vi "ViperHawk_Decode Inv Data.vi"(9 "Washer In":T1={"Appliance Details"={"FileVersionInfo"={"FileVersion"="Version", "ProductName"="ProductName", "InternalName"="InternalName", "CompanyName"="CompanyName", "LegalCopyright"="LegalCopyright", "FileDescription"="FileDescription"}, "Dishwasher Info"={"Open Cup Weight (gm):"=0.0, "Auto Cup Weight (gm):"=0.0, "Detergent-Dish:"="", "Inlet Temperature-Dish:"="", "Cycle Mode-Dish:"="", "Unit Control-Dish:"="", "Manufacturer-Dish:"=""}, "Washer Info"={"Hot Water Temperature (Fahrenheit):"="", "Cold Water Temperature (Fahrenheit):"="", "Capacity (cu.ft):"=0.0, "Initial Cloth Weight:"=0.0, "Cloth Lot:"=0, "Model Family:"="", "Program Name:"="", "Cycle Selection:"="", "Wash Temperature:"="", "Rinse Temperature:"="", "Load Size:"=""}, "File Name Output Array"=[], "Calibration Output Array"=[], "Appliance Common"={"Engineer:"="", "Model Number:"="", "Serial Number:"="15HL2790", "Comments:"="", "Station ID:"="", "Technician:"="", "TR Number:"="15HL2790", "Lab ID:"="15HL2790", "Voltage:"="", "Water Pressure (PSI):"="", "Test Date:"="", "Computer Name:"="", "IP Address:"="", "Ambient RH:"="", "Frequency:"="", "Build:"="", "Filename:"="", "Test Type:"="", "Load Run #:"=0, "Ambient Temperature (F):"="", "File Path:"=path "", "Cycles Per Year"=60}, "Water Heater"={"Heating Mode:"=""}, "Dryer"={"Heat Setting:"="", "Washer Water Temperature (60 ± 5°F):"=60, "Water Hardness (PPM):"=17, "Dryness Setting:"="", "Dryer Type:"="", "Exhaust:"="", "Drying Cycle:"="", "Load Type:"="", "Nominal Load Weight"="", "Dryer Initial IMC Data"={"Measured IMC (lbs)"=7.0, "Actual Initial RMC (%)"=7.0, "RMC (Desired %)"=100.0, "Bone Dry Wt(lbs)"=7.0, "Tolerance(%)"=5.0, "Actual Final RMC (%)"=7.0, "CEF (lbf/kWh)"=0.0, "Minimum Weight (lbf)"=0.0, "Average Weight (lbf)"=0.0, "Maximum Weight (lbf)"=0.0, "Measured IMC In Range?"=FALSE, "Moisture Reduction Factor"=55.5, "Field Use Factor"=1.04, "Empty Dryer Cold Weigth"=0.0, "Energy Standard"=enum."D2-Automatic Dryer", "Weight Cloth (lbs)"=0.0, "Relative Moisture Content (%)"=0.0, "Relative Moisture Content - Avg (%)"=0.0}}}, "Display Data (RLT)"={"Status Color"=14927872, "Serial Number Display"="15HL2790", "Cycle Count Display"=0, "Station Label Display"="04125059", "Current Run Start Time Display"=0.0, "Board ID Display"="", "RPM Display"=0, "Current Display"=1.0, "Current Path Display"=path "", "Saving Display"=FALSE, "Unit Type Display"=enum."2015", "Total Time On Display"=0.0, "UI Button"=FALSE}} {"Display Data (RLT)"."Current Display" format="%.2f"; "Display Data (RLT)"."Cycle Count Display" format="%04d"; "Appliance Details"."Dryer"."Dryer Initial IMC Data"."Maximum Weight (lbf)" format="%03_6g"; "Appliance Details"."Dryer"."Dryer Initial IMC Data"."Average Weight (lbf)" format="%03_6g"; "Appliance Details"."Dryer"."Dryer Initial IMC Data"."Minimum Weight (lbf)" format="%03_6g"; "Appliance Details"."Dryer"."Dryer Initial IMC Data"."CEF (lbf/kWh)" format="%03_6g"; "Appliance Details"."Dryer"."Dryer Initial IMC Data"."Actual Final RMC (%)" format="%03_6g"; "Appliance Details"."Dryer"."Dryer Initial IMC Data"."Tolerance(%)" format="%0#_6g"; "Appliance Details"."Dryer"."Dryer Initial IMC Data"."Bone Dry Wt(lbs)" format="%03_6g"; "Appliance Details"."Dryer"."Dryer Initial IMC Data"."RMC (Desired %)" format="%0#_6g"; "Appliance Details"."Dryer"."Dryer Initial IMC Data"."Actual Initial RMC (%)" format="%03_6g"; "Appliance Details"."Dryer"."Dryer Initial IMC Data"."Measured IMC (lbs)" format="%0#_6g"}, 10 "Data":u8[](array[numeric]), 11 "Diagnostic Data In":T10) -> (1 "Washer Out":T1={"Appliance Details"={"FileVersionInfo"={"FileVersion"="Version", "ProductName"="ProductName", "InternalName"="InternalName", "CompanyName"="CompanyName", "LegalCopyright"="LegalCopyright", "FileDescription"="FileDescription"}, "Dishwasher Info"={"Open Cup Weight (gm):"=0.0, "Auto Cup Weight (gm):"=0.0, "Detergent-Dish:"="", "Inlet Temperature-Dish:"="", "Cycle Mode-Dish:"="", "Unit Control-Dish:"="", "Manufacturer-Dish:"=""}, "Washer Info"={"Hot Water Temperature (Fahrenheit):"="", "Cold Water Temperature (Fahrenheit):"="", "Capacity (cu.ft):"=0.0, "Initial Cloth Weight:"=0.0, "Cloth Lot:"=0, "Model Family:"="", "Program Name:"="", "Cycle Selection:"="", "Wash Temperature:"="", "Rinse Temperature:"="", "Load Size:"=""}, "File Name Output Array"=[], "Calibration Output Array"=[], "Appliance Common"={"Engineer:"="", "Model Number:"="", "Serial Number:"="15HL2790", "Comments:"="", "Station ID:"="", "Technician:"="", "TR Number:"="15HL2790", "Lab ID:"="15HL2790", "Voltage:"="", "Water Pressure (PSI):"="", "Test Date:"="", "Computer Name:"="", "IP Address:"="", "Ambient RH:"="", "Frequency:"="", "Build:"="", "Filename:"="", "Test Type:"="", "Load Run #:"=0, "Ambient Temperature (F):"="", "File Path:"=path "", "Cycles Per Year"=60}, "Water Heater"={"Heating Mode:"=""}, "Dryer"={"Heat Setting:"="", "Washer Water Temperature (60 ± 5°F):"=60, "Water Hardness (PPM):"=17, "Dryness Setting:"="", "Dryer Type:"="", "Exhaust:"="", "Drying Cycle:"="", "Load Type:"="", "Nominal Load Weight"="", "Dryer Initial IMC Data"={"Measured IMC (lbs)"=7.0, "Actual Initial RMC (%)"=7.0, "RMC (Desired %)"=100.0, "Bone Dry Wt(lbs)"=7.0, "Tolerance(%)"=5.0, "Actual Final RMC (%)"=7.0, "CEF (lbf/kWh)"=0.0, "Minimum Weight (lbf)"=0.0, "Average Weight (lbf)"=0.0, "Maximum Weight (lbf)"=0.0, "Measured IMC In Range?"=FALSE, "Moisture Reduction Factor"=55.5, "Field Use Factor"=1.04, "Empty Dryer Cold Weigth"=0.0, "Energy Standard"=enum."D2-Automatic Dryer", "Weight Cloth (lbs)"=0.0, "Relative Moisture Content (%)"=0.0, "Relative Moisture Content - Avg (%)"=0.0}}}, "Display Data (RLT)"={"Status Color"=14927872, "Serial Number Display"="15HL2790", "Cycle Count Display"=0, "Station Label Display"="04125059", "Current Run Start Time Display"=0.0, "Board ID Display"="", "RPM Display"=0, "Current Display"=1.0, "Current Path Display"=path "", "Saving Display"=FALSE, "Unit Type Display"=enum."2015", "Total Time On Display"=0.0, "UI Button"=FALSE}} {"Display Data (RLT)"."Current Display" format="%.2f"; "Display Data (RLT)"."Cycle Count Display" format="%04d"; "Appliance Details"."Dryer"."Dryer Initial IMC Data"."Maximum Weight (lbf)" format="%03_6g"; "Appliance Details"."Dryer"."Dryer Initial IMC Data"."Average Weight (lbf)" format="%03_6g"; "Appliance Details"."Dryer"."Dryer Initial IMC Data"."Minimum Weight (lbf)" format="%03_6g"; "Appliance Details"."Dryer"."Dryer Initial IMC Data"."CEF (lbf/kWh)" format="%03_6g"; "Appliance Details"."Dryer"."Dryer Initial IMC Data"."Actual Final RMC (%)" format="%03_6g"; "Appliance Details"."Dryer"."Dryer Initial IMC Data"."Tolerance(%)" format="%0#_6g"; "Appliance Details"."Dryer"."Dryer Initial IMC Data"."Bone Dry Wt(lbs)" format="%03_6g"; "Appliance Details"."Dryer"."Dryer Initial IMC Data"."RMC (Desired %)" format="%0#_6g"; "Appliance Details"."Dryer"."Dryer Initial IMC Data"."Actual Initial RMC (%)" format="%03_6g"; "Appliance Details"."Dryer"."Dryer Initial IMC Data"."Measured IMC (lbs)" format="%0#_6g"}, 2 "Value":u8 format="%.0x", 3 "Diagnostic Data Out":T10)   [LabVIEW 2016]
uses:
  Type Definitions/ViperHawk/ViperHawk Diagnostic Data.ctl
  Utility/Save File/Public/Type Definitions/Save File Washer.ctl
  Utility/Save File/File Setup (Public)/Type Definition/Save File DISH Dishwasher Details.ctl
  <vilib>/Platform/fileVersionInfo.llb/FileVersionInformation.ctl
  Washer DOE/Type Definitions/DOE Appliance Common.ctl
  Utility/Custom Pallet Controls/Custom Pallet String.ctl
  Utility/Save File/File Setup (Public)/Type Definition/DPT IMC Data.ctl
  Washer DOE/Type Definitions/DOE Dryer Standard.ctl
  Utility/Save File/Public/Type Definitions/Save File Appliance Display.ctl
  Utility/Save File/Public/Type Definitions/Save File Unit Type.ctl
  Utility/LabVIEW GEA2 Toolkit v1.0.0.0/library/GEA2_Toolkit.lvlib
  Utility/Save File/Save File.lvlib
  Utility/Save File/File Setup.lvlib
panel:
  in  "string":string
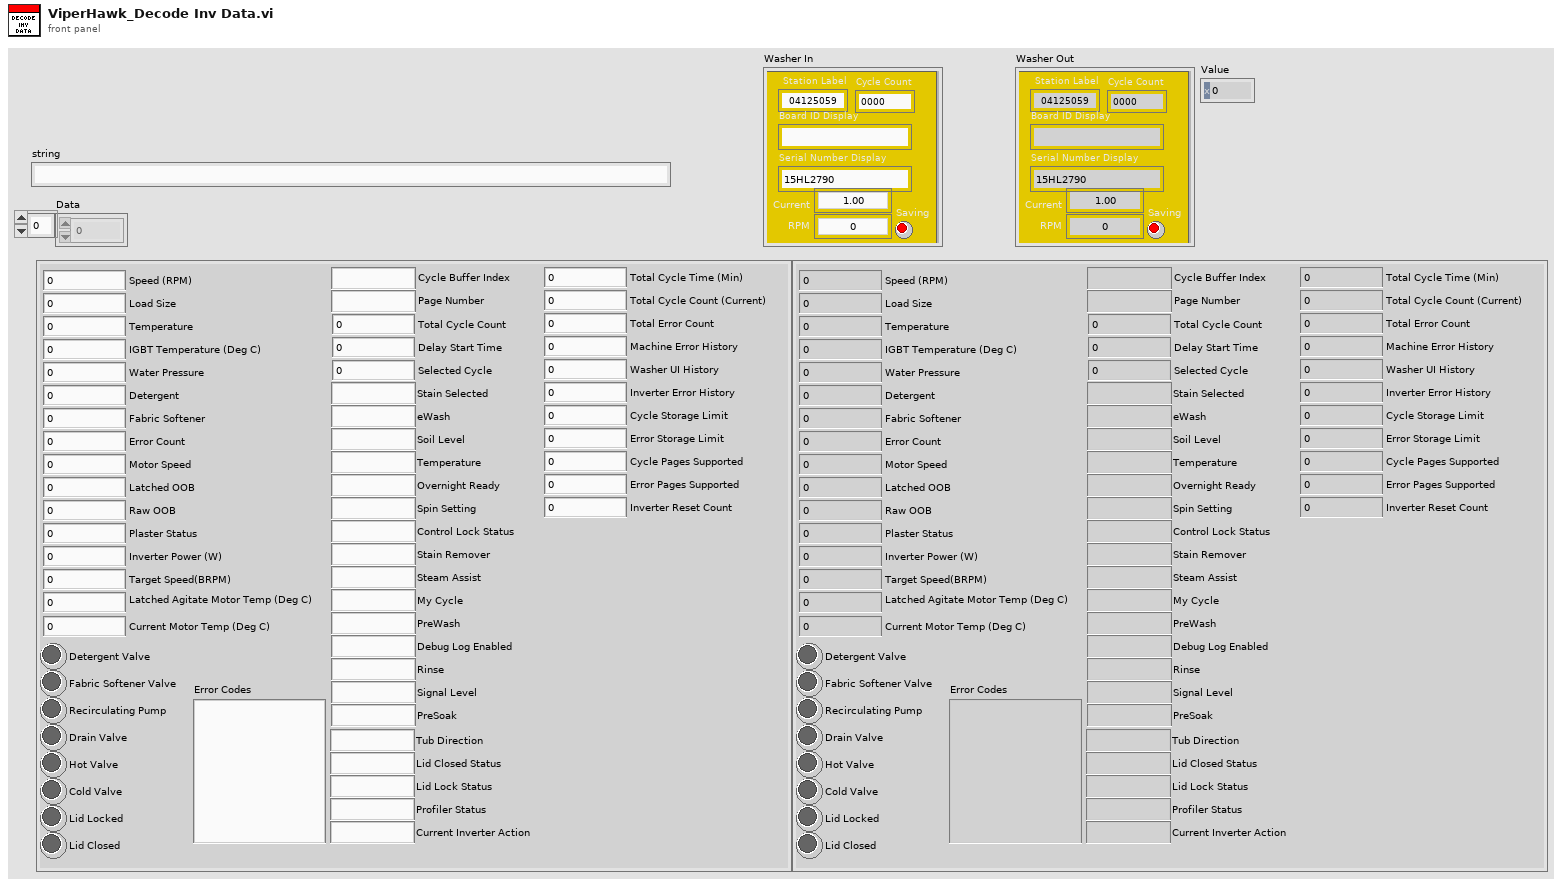
[diagram p1: front panel]
types:
  T1 = typedef "Save File.lvlib/Save File Washer.ctl" = cluster{"Appliance Details":T2, "Display Data (RLT)":T8}
  T2 = typedef "File Setup.lvlib/Save File DISH Dishwasher Details.ctl" = cluster{"FileVersionInfo":T3, "Dishwasher Info":cluster{"Open Cup Weight (gm):":dbl, "Auto Cup Weight (gm):":dbl, "Detergent-Dish:":string, "Inlet Temperature-Dish:":string, "Cycle Mode-Dish:":string, "Unit Control-Dish:":string, "Manufacturer-Dish:":string}, "Washer Info":cluster{"Hot Water Temperature (Fahrenheit):":string, "Cold Water Temperature (Fahrenheit):":string, "Capacity (cu.ft):":dbl, "Initial Cloth Weight:":dbl, "Cloth Lot:":i32, "Model Family:":string, "Program Name:":string, "Cycle Selection:":string, "Wash Temperature:":string, "Rinse Temperature:":string, "Load Size:":string}, "File Name Output Array":string[][], "Calibration Output Array":string[][], "Appliance Common":T4, "Water Heater":cluster{"Heating Mode:":string}, "Dryer":cluster{"Heat Setting:":T5, "Washer Water Temperature (60 ± 5°F):":u16, "Water Hardness (PPM):":u16, "Dryness Setting:":T5, "Dryer Type:":string, "Exhaust:":string, "Drying Cycle:":string, "Load Type:":string, "Nominal Load Weight":string, "Dryer Initial IMC Data":T6}}
  T3 = typedef "FileVersionInformation.ctl" = cluster{"FileVersion":string, "ProductName":string, "InternalName":string, "CompanyName":string, "LegalCopyright":string, "FileDescription":string}
  T4 = typedef "DOE Appliance Common.ctl" = cluster{"Engineer:":string, "Model Number:":string, "Serial Number:":string, "Comments:":string, "Station ID:":string, "Technician:":string, "TR Number:":string, "Lab ID:":string, "Voltage:":string, "Water Pressure (PSI):":string, "Test Date:":string, "Computer Name:":string, "IP Address:":string, "Ambient RH:":string, "Frequency:":string, "Build:":string, "Filename:":string, "Test Type:":string, "Load Run #:":i32, "Ambient Temperature (F):":string, "File Path:":path, "Cycles Per Year":u32}
  T5 = typedef "Custom Pallet String.ctl" = string
  T6 = typedef "DPT IMC Data.ctl" = cluster{"Measured IMC (lbs)":dbl, "Actual Initial RMC (%)":dbl, "RMC (Desired %)":dbl, "Bone Dry Wt(lbs)":dbl, "Tolerance(%)":dbl, "Actual Final RMC (%)":dbl, "CEF (lbf/kWh)":dbl, "Minimum Weight (lbf)":dbl, "Average Weight (lbf)":dbl, "Maximum Weight (lbf)":dbl, "Measured IMC In Range?":bool, "Moisture Reduction Factor":dbl, "Field Use Factor":dbl, "Empty Dryer Cold Weigth":dbl, "Energy Standard":T7, "Weight Cloth (lbs)":dbl, "Relative Moisture Content (%)":dbl, "Relative Moisture Content - Avg (%)":dbl}
  T7 = typedef "DOE Dryer Standard.ctl" = enum16{"D2-Automatic Dryer", "D2-Timer Dryer", "D1-Automatic Dryer", "D1-Timer Dryer", "Other"}
  T8 = typedef "Save File Appliance Display.ctl" = cluster{"Status Color":u32, "Serial Number Display":string, "Cycle Count Display":i32, "Station Label Display":string, "Current Run Start Time Display":dbl, "Board ID Display":string, "RPM Display":u32, "Current Display":dbl, "Current Path Display":path, "Saving Display":bool, "Unit Type Display":T9, "Total Time On Display":dbl, "UI Button":bool}
  T9 = typedef "Save File.lvlib/Save File Unit Type.ctl" = enum32{"", "Viper", "Hawk", "2015"}
  T10 = typedef "ViperHawk Diagnostic Data.ctl" = cluster{"Speed (RPM)":u32, "Load Size":u32, "Temperature":u32, "Water Pressure":dbl, "Detergent":u32, "Fabric Softener":u32, "Tub Direction":string, "Detergent Valve":bool, "Fabric Softener Valve":bool, "Recirculating Pump":bool, "Drain Valve":bool, "Hot Valve":bool, "Cold Valve":bool, "Lid Closed Status":string, "Lid Lock Status":string, "Error Count":u32, "IGBT Temperature (Deg C)":u32, "Motor Speed":u32, "Latched OOB":u32, "Raw OOB":u32, "Plaster Status":u32, "Inverter Power (W)":u32, "Target Speed(BRPM)":u32, "Latched Agitate Motor Temp (Deg C)":u32, "Current Motor Temp (Deg C)":u32, "Profiler Status":string, "Current Inverter Action":string, "Error Codes":string, "Lid Locked":bool, "Lid Closed":bool, "9E Diagnostic Data":cluster{"Total Cycle Time (Min)":u32, "Total Cycle Count (Current)":u16, "Total Error Count":u16, "Machine Error History":u32, "Washer UI History":u32, "Inverter Error History":u32, "Cycle Storage Limit":u8, "Error Storage Limit":u8, "Cycle Pages Supported":u8, "Error Pages Supported":u8, "Inverter Reset Count":u16}, "9F Diagnostic Data":cluster{"Cycle Buffer Index":string, "Page Number":string, "Total Cycle Count":u32, "Delay Start Time":u32, "Stain Selected":string, "Selected Cycle":u32, "eWash":string, "Soil Level":string, "Temperature":string, "Overnight Ready":string, "Spin Setting":string, "Control Lock Status":string, "Stain Remover":string, "Steam Assist":string, "My Cycle":string, "PreWash":string, "Debug Log Enabled":string, "Rinse":string, "Signal Level":string, "PreSoak":string}}
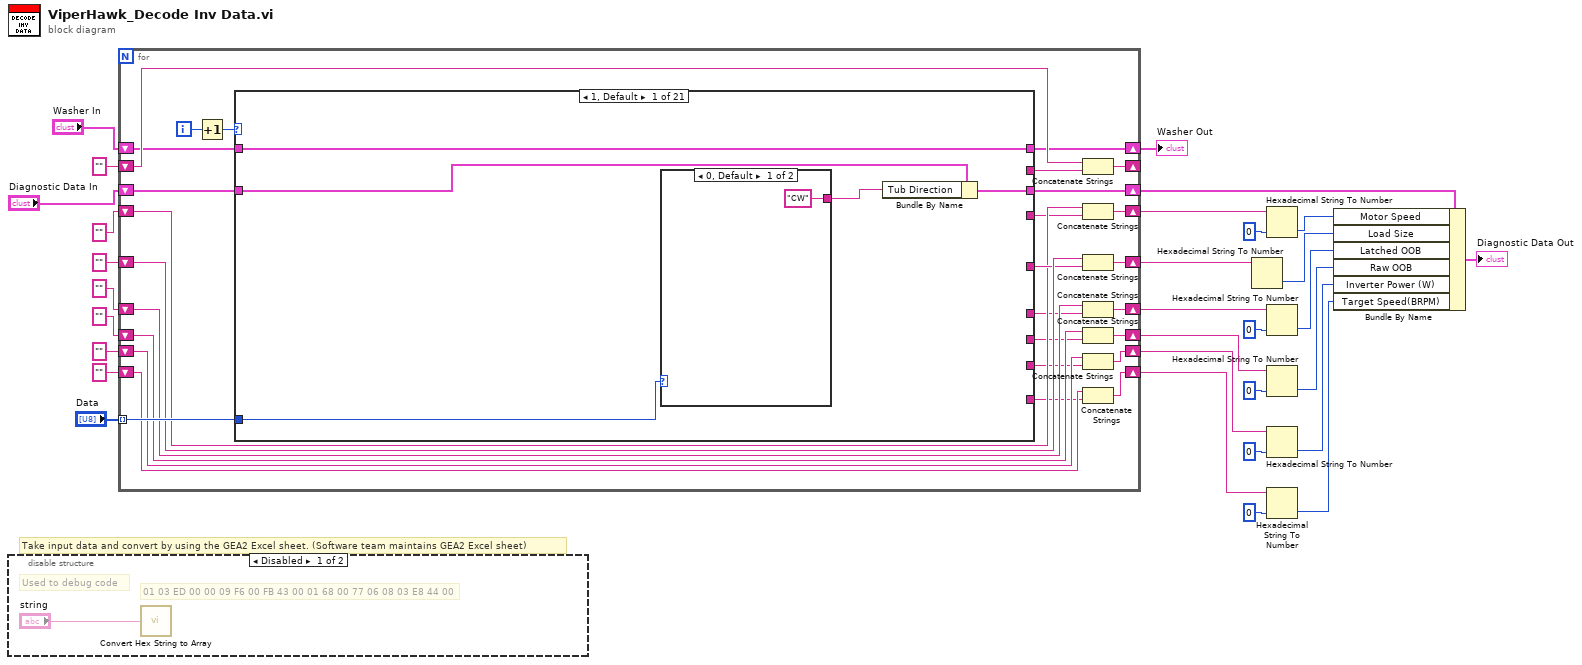
[diagram p0: block diagram]
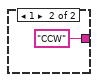
[diagram p3: hidden frame]
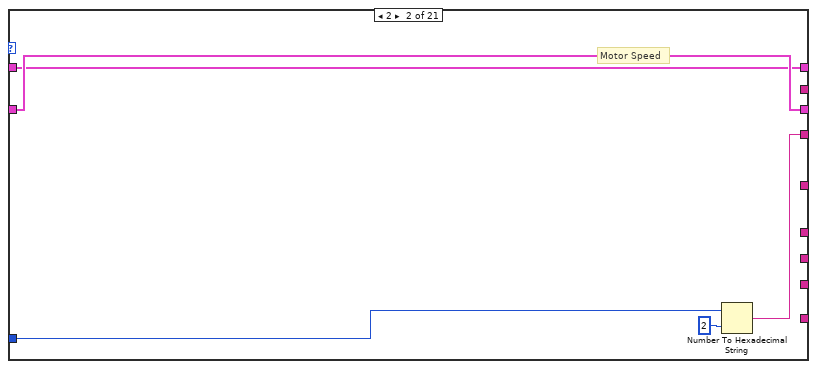
[diagram p4: hidden frame]
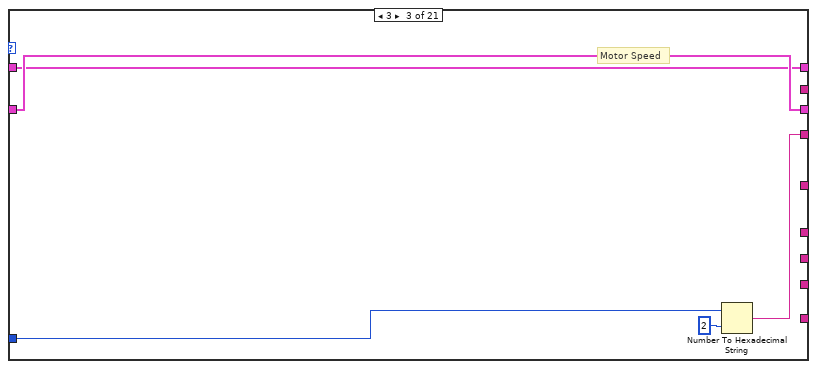
[diagram p5: hidden frame]
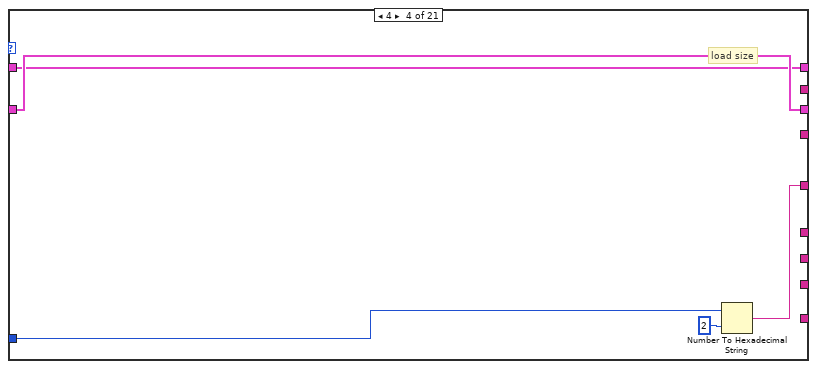
[diagram p6: hidden frame]
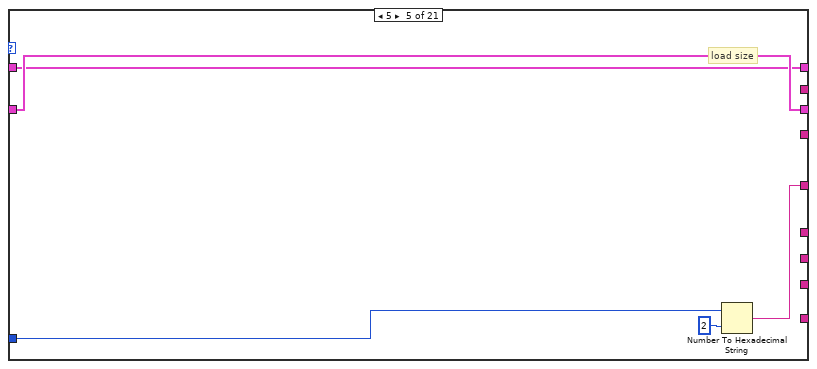
[diagram p7: hidden frame]
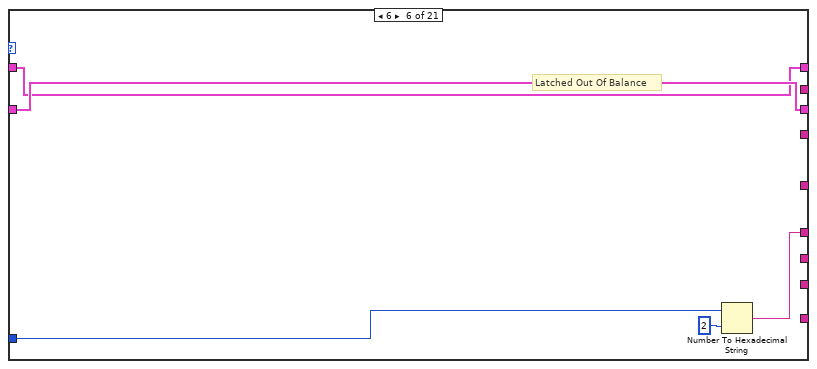
[diagram p8: hidden frame]
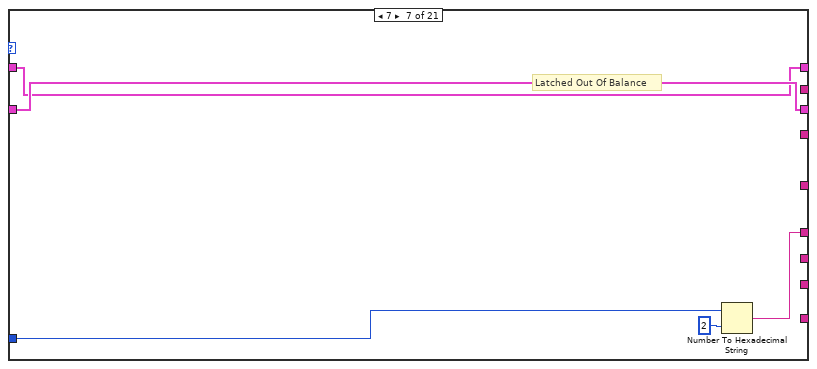
[diagram p9: hidden frame]
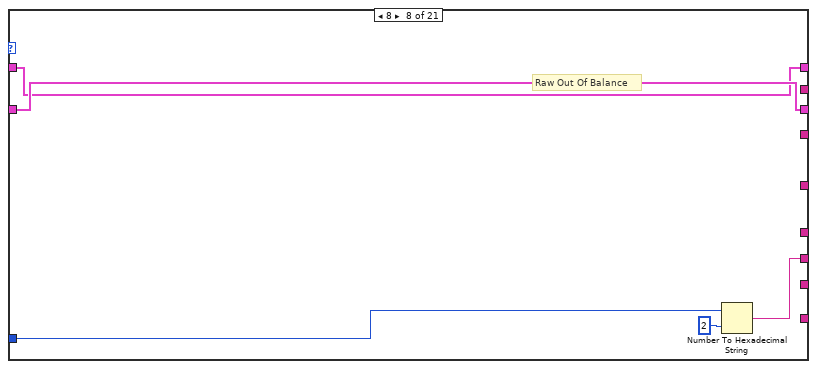
[diagram p10: hidden frame]
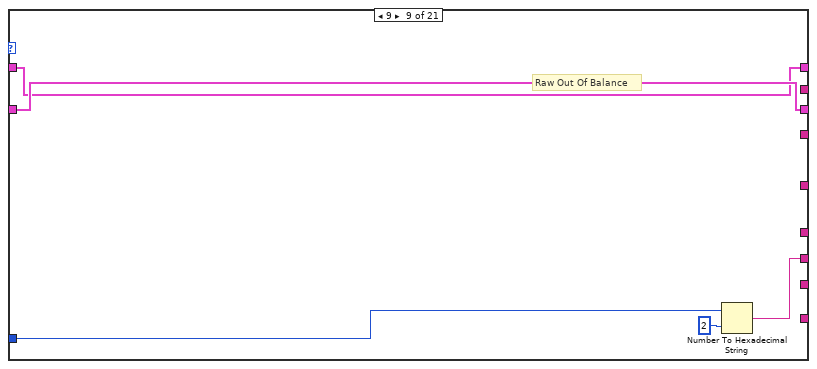
[diagram p11: hidden frame]
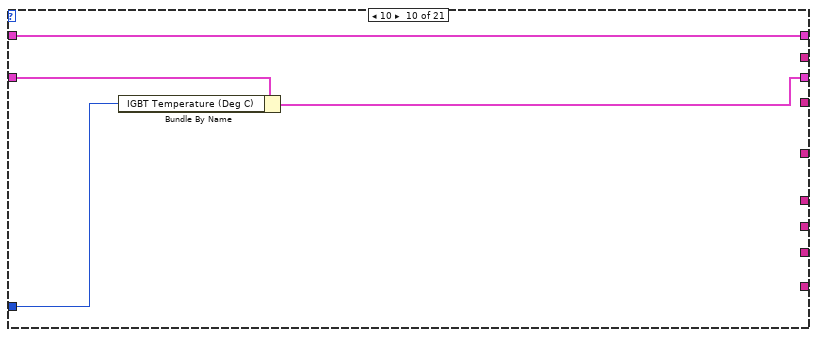
[diagram p12: hidden frame]
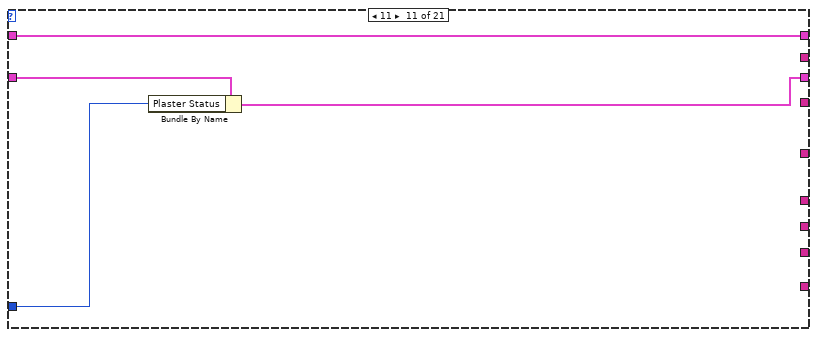
[diagram p13: hidden frame]
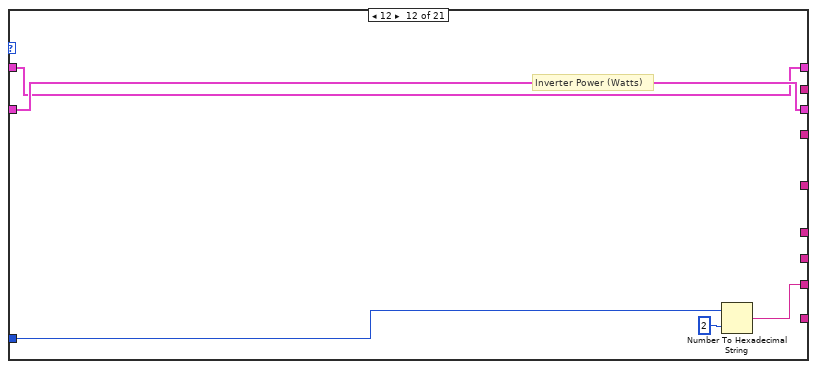
[diagram p14: hidden frame]
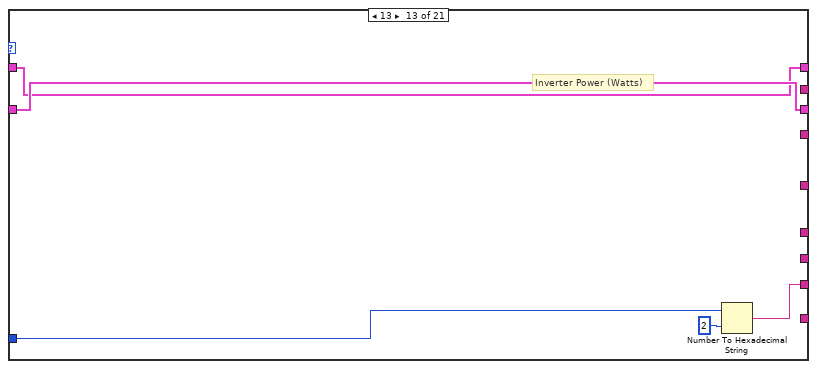
[diagram p15: hidden frame]
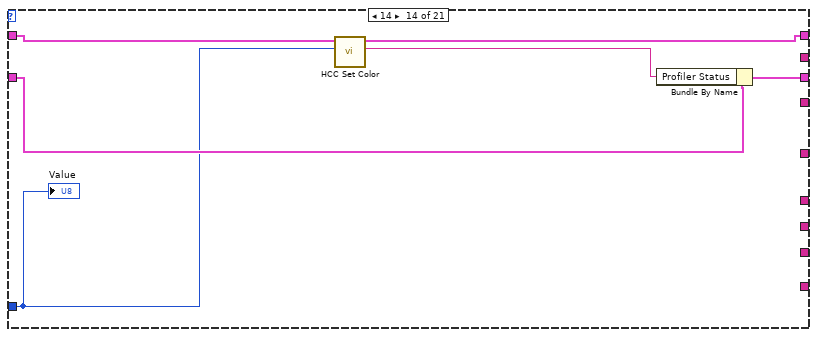
[diagram p16: hidden frame]
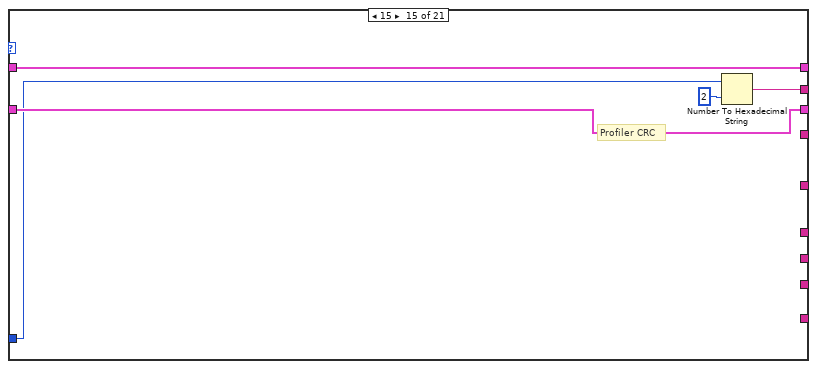
[diagram p17: hidden frame]
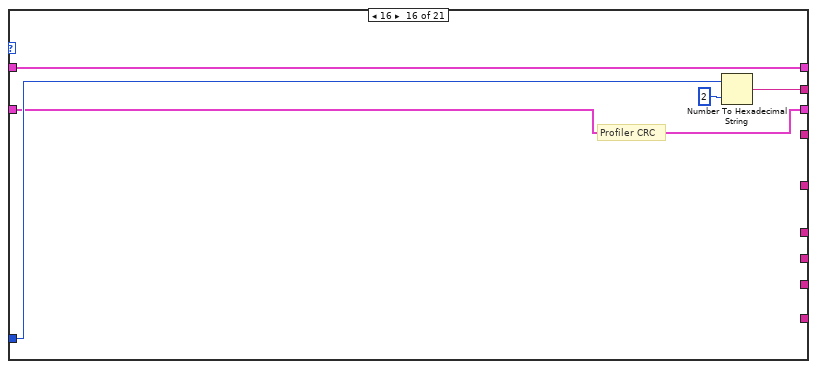
[diagram p18: hidden frame]
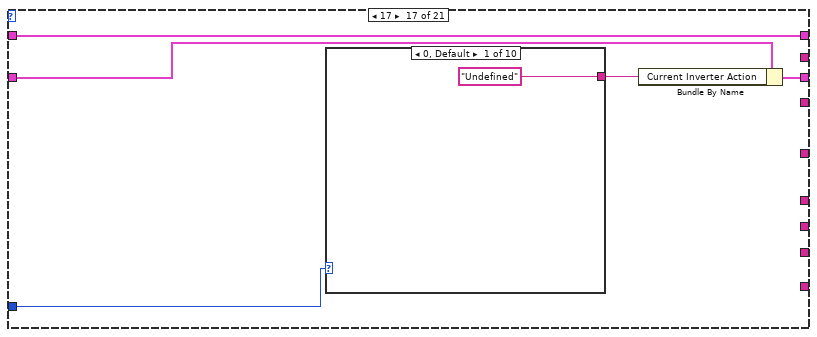
[diagram p19: hidden frame]
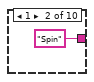
[diagram p20: hidden frame]
diagram:
  # "Take input data and convert by using the GEA2 Excel sheet. (Software team maintains GEA2 Excel sheet)"
  n1 = disable-structure shown="Disabled" {
    frame Disabled {
      # "01 03 ED 00 00 09 F6 00 FB 43 00 01 68 00 77 06 08 03 E8 44 00"
      # "Used to debug code"
      n2 = call "Convert Hex String to Array.vi"("Hex String In"="string") -> ()  [unwired: 14 in, 1 out]
    }
    frame Enabled {
    }
  }
  n3 = for {
    tunnel: "Data" -> [w59] mode=indexing
    shift-right: [w57] -> w29
    shift-left: "" -> [w56]
    shift-right: [w55] -> w30
    shift-left: "Diagnostic Data In" -> [w54]
    shift-right: [w49] -> w25
    shift-left: "" -> [w51]
    shift-right: [w46] -> w21
    shift-left: "" -> [w48]
    shift-right: [w43] -> w16
    shift-left: "" -> [w45]
    shift-right: [w40] -> w12
    shift-left: "" -> [w42]
    shift-right: [w37] -> _
    shift-left: "" -> [w39]
    shift-right: [w34] -> w7
    shift-left: "" -> [w36]
    shift-right: [w32] -> w2
    shift-left: "Washer In" -> [w33]
    i -> [w58]
    n4 = Increment(x=w58) -> (x+1=w53:i32)
    n5 = case shown="1, Default" w53 {
      tunnel: w59 -> [w64 w70 w75 w81 w85 w90 w95 w101 w105 w108 w112 w118 w123 w128 w134 w140 w143 w159 w164 w167 w171]
      tunnel: [_ _ _ w80 w86 _ _ _ _ _ _ _ _ _ _ _ _ _ _ _ _] -> w52
      tunnel: w54 -> [w63 w71 w76 w79 w84 w91 w96 w100 w106 w110 w114 w119 w124 w130 w135 w139 w145 w160 w165 w169 w173]
      tunnel: [w62 w71 w76 w79 w84 w91 w96 w100 w106 w109 w113 w119 w124 w129 w135 w139 w144 w160 w165 w168 w172] -> w55
      tunnel: [_ w69 w74 _ _ _ _ _ _ _ _ _ _ _ _ _ _ _ _ _ _] -> w50
      tunnel: [_ _ _ _ _ w89 w94 _ _ _ _ _ _ _ _ _ _ _ _ _ _] -> w47
      tunnel: [_ _ _ _ _ _ _ w99 w104 _ _ _ _ _ _ _ _ _ _ _ _] -> w44
      tunnel: [_ _ _ _ _ _ _ _ _ _ _ w117 w122 _ _ _ _ _ _ _ _] -> w41
      tunnel: [_ _ _ _ _ _ _ _ _ _ _ _ _ _ w133 w138 _ _ _ _ _] -> w38
      tunnel: [_ _ _ _ _ _ _ _ _ _ _ _ _ _ _ _ _ w158 w163 _ _] -> w35
      tunnel: w33 -> [w60 w67 w72 w77 w82 w87 w92 w97 w102 w107 w111 w115 w120 w126 w131 w136 w141 w156 w161 w166 w170]
      tunnel: [w60 w67 w72 w77 w82 w87 w92 w97 w102 w107 w111 w115 w120 w125 w131 w136 w141 w156 w161 w166 w170] -> w32
      frame 1, Default {
        n6 = case shown="0, Default" w64 {
          tunnel: ["CW" ("String") "CCW" ("String")] -> w61
          frame 0, Default {
          }
          frame 1 {
          }
        }
        n7 = Bundle By Name(cluster=w63, "Tub Direction"=w61) -> (w62:T10)
      }
      frame 2 {
        # "Motor Speed"
        n8 = Number To Hexadecimal String(1:i16 2 ("width (-)"), 2:w70) -> (0:w69:string)
      }
      frame 3 {
        # "Motor Speed"
        n9 = Number To Hexadecimal String(1:i16 2 ("width (-)"), 2:w75) -> (0:w74:string)
      }
      frame 4 {
        # "load size"
        n10 = Number To Hexadecimal String(1:i16 2 ("width (-)"), 2:w81) -> (0:w80:string)
      }
      frame 5 {
        # "load size"
        n11 = Number To Hexadecimal String(1:i16 2 ("width (-)"), 2:w85) -> (0:w86:string)
      }
      frame 6 {
        # "Latched Out Of Balance"
        n12 = Number To Hexadecimal String(1:i16 2 ("width (-)"), 2:w90) -> (0:w89:string)
      }
      frame 7 {
        # "Latched Out Of Balance"
        n13 = Number To Hexadecimal String(1:i16 2 ("width (-)"), 2:w95) -> (0:w94:string)
      }
      frame 8 {
        # "Raw Out Of Balance"
        n14 = Number To Hexadecimal String(1:i16 2 ("width (-)"), 2:w101) -> (0:w99:string)
      }
      frame 9 {
        # "Raw Out Of Balance"
        n15 = Number To Hexadecimal String(1:i16 2 ("width (-)"), 2:w105) -> (0:w104:string)
      }
      frame 10 {
        n16 = Bundle By Name(cluster=w110, "IGBT Temperature (Deg C)"=w108) -> (w109:T10)
      }
      frame 11 {
        n17 = Bundle By Name(cluster=w114, "Plaster Status"=w112) -> (w113:T10)
      }
      frame 12 {
        # "Inverter Power (Watts)"
        n18 = Number To Hexadecimal String(1:i16 2 ("width (-)"), 2:w118) -> (0:w117:string)
      }
      frame 13 {
        # "Inverter Power (Watts)"
        n19 = Number To Hexadecimal String(1:i16 2 ("width (-)"), 2:w123) -> (0:w122:string)
      }
      frame 14 {
        n20 = call "HCC Set Color.vi"("Value"=w128, "Washer In in"=w126) -> ("String"=w127:string, "Washer In out"=w125:T1)  [unwired: 8 in]
        n21 = Bundle By Name(cluster=w130, "Profiler Status"=w127) -> (w129:T10)
        "Value" <- w128
      }
      frame 15 {
        # "Profiler CRC"
        n22 = Number To Hexadecimal String(1:i16 2 ("width (-)"), 2:w134) -> (0:w133:string)
      }
      frame 16 {
        # "Profiler CRC"
        n23 = Number To Hexadecimal String(1:i16 2 ("width (-)"), 2:w140) -> (0:w138:string)
      }
      frame 17 {
        n24 = case shown="0, Default" w143 {
          tunnel: ["Undefined" "Spin" "Coast" "Brake" "OOB" "Load Sense" "Position" "Inertia Test" "ATW" "Profiler"] -> w142
          frame 0, Default {
          }
          frame 1 {
          }
          frame 2 {
          }
          frame 3 {
          }
          frame 4 {
          }
          frame 5 {
          }
          frame 6 {
          }
          frame 7 {
          }
          frame 8 {
          }
          frame 9 {
          }
        }
        n25 = Bundle By Name(cluster=w145, "Current Inverter Action"=w142) -> (w144:T10)
      }
      frame 18 {
        # "Target Speed"
        n26 = Number To Hexadecimal String(1:i16 2 ("width (-)"), 2:w159) -> (0:w158:string)
      }
      frame 19 {
        # "Target Speed"
        n27 = Number To Hexadecimal String(1:i16 2 ("width (-)"), 2:w164) -> (0:w163:string)
      }
      frame 20 {
        n28 = Bundle By Name(cluster=w169, "Latched Agitate Motor Temp (Deg C)"=w167) -> (w168:T10)
      }
      frame 21 {
        n29 = Bundle By Name(cluster=w173, "Current Motor Temp (Deg C)"=w171) -> (w172:T10)
      }
    }
    n30 = Concatenate Strings(w39, w38) -> (w37:string)
    n31 = Concatenate Strings(w51, w50) -> (w49:string)
    n32 = Concatenate Strings(w56, w52) -> (w57:string)
    n33 = Concatenate Strings(w48, w47) -> (w46:string)
    n34 = Concatenate Strings(w45, w44) -> (w43:string)
    n35 = Concatenate Strings(w42, w41) -> (w40:string)
    n36 = Concatenate Strings(w36, w35) -> (w34:string)
  }
  "Washer Out" <- w2
  n37 = Hexadecimal String To Number(string=w29) -> (number=w22:u32)  [unwired: 2 in, 1 out]
  n38 = Hexadecimal String To Number(string=w25, default (0uL)=u16 0 ("default (0 U32)")) -> (number=w27:u16)  [unwired: 1 in, 1 out]
  n39 = Hexadecimal String To Number(string=w21, default (0uL)=u16 0 ("default (0 U32)")) -> (number=w20:u16)  [unwired: 1 in, 1 out]
  n40 = Hexadecimal String To Number(string=w16, default (0uL)=u16 0 ("default (0 U32)")) -> (number=w15:u16)  [unwired: 1 in, 1 out]
  n41 = Hexadecimal String To Number(string=w12, default (0uL)=u16 0 ("default (0 U32)")) -> (number=w11:u16)  [unwired: 1 in, 1 out]
  n42 = Hexadecimal String To Number(string=w7, default (0uL)=u16 0 ("default (0 U32)")) -> (number=w6:u16)  [unwired: 1 in, 1 out]
  n43 = Bundle By Name(cluster=w30, "Motor Speed"=w27, "Load Size"=w22, "Latched OOB"=w20, "Raw OOB"=w15, "Inverter Power (W)"=w11, "Target Speed(BRPM)"=w6) -> (→"Diagnostic Data Out":T10)
